vi "All Square1.vi"() -> ()   [LabVIEW 2023]
panel:
  in  "Stop 7":bool
  in  "Stop 6":bool
  in  "Stop 5":bool
  in  "Stop 4":bool
  in  "Stop 3":bool
  in  "Stop 2":bool
  in  "Start 2":bool
  in  "Start":bool
  in  "Remove 4":bool
  in  "Remove 3":bool
  in  "Remove 2":bool
  in  "Remove":bool
  in  "OK 5":bool
  in  "OK 4":bool
  in  "OK 3":bool
  in  "OK 2":bool
  in  "OK":bool
  in  "Hibernet":bool
  in  "Halt":bool
  in  "Finish 4":bool
  in  "Finish 3":bool
  in  "Finish 2":bool
  in  "Finish":bool
  in  "Exit 5":bool
  in  "Exit 4":bool
  in  "Exit 3":bool
  in  "Exit 2":bool
  in  "Exit":bool
  in  "EXE":bool
  in  "Delete 2":bool
  in  "Delete":bool
  in  "Close 4":bool
  in  "Close 3":bool
  in  "Close 2":bool
  in  "Close":bool
  in  "Clear":bool
  in  "Cancel 4":bool
  in  "Cancel 3":bool
  in  "Cancel 2":bool
  in  "Cancel":bool
  in  "Apply 7":bool
  in  "Apply 6":bool
  in  "Apply 5":bool
  in  "Apply 4":bool
  in  "Apply 3":bool
  in  "Apply 2":bool
  in  "Apply":bool
  in  "Add 6":bool
  in  "Add 5":bool
  in  "Add 4":bool
  in  "Add 3":bool
  in  "Add 2":bool
  in  "Add":bool
  in  "Stop":bool
  in  "DB_Remove":bool
  in  "DB_Comit":bool
  in  "DB_Add":bool
  in  "URL":bool
  in  "UP 7":bool
  in  "UP 6":bool
  in  "UP 5":bool
  in  "UP 4":bool
  in  "UP 3":bool
  in  "UP 2":bool
  in  "UP":bool
  in  "Undo 2":bool
  in  "Undo":bool
  in  "Top 3":bool
  in  "Top 2":bool
  in  "Top":bool
  in  "Reload 2":bool
  in  "Reload":bool
  in  "Refresh 3":bool
  in  "Refresh 2":bool
  in  "Refresh":bool
  in  "Redo 2":bool
  in  "Redo":bool
  in  "Next 8":bool
  in  "Next 7":bool
  in  "Next 6":bool
  in  "Next 5":bool
  in  "Next 4":bool
  in  "Next 3":bool
  in  "Next 2":bool
  in  "Next":bool
  in  "Exchange":bool
  in  "Down 7":bool
  in  "Down 6":bool
  in  "Down 5":bool
  in  "Down 4":bool
  in  "Down 3":bool
  in  "Down 2":bool
  in  "Down":bool
  in  "Bottom 4":bool
  in  "Bottom 3":bool
  in  "Bottom 2":bool
  in  "Bottom":bool
  in  "Back 9":bool
  in  "Back 8":bool
  in  "Back 7":bool
  in  "Back 6":bool
  in  "Back 5":bool
  in  "Back 4":bool
  in  "Back 3":bool
  in  "Back 2":bool
  in  "Back":bool
  in  "XML":bool
  in  "Word":bool
  in  "Text":bool
  in  "Sync":bool
  in  "SQL":bool
  in  "PPT":bool
  in  "PNG 2":bool
  in  "PNG":bool
  in  "Play 4":bool
  in  "PDF 4":bool
  in  "PDF 3":bool
  in  "PDF 2":bool
  in  "PDF":bool
  in  "Paint":bool
  in  "Notepad":bool
  in  "JPG":bool
  in  "JPEG 2":bool
  in  "JPEG":bool
  in  "Java":bool
  in  "Jar":bool
  in  "GIF":bool
  in  "Excel":bool
  in  "Docs":bool
  in  "CHM":bool
  in  "C++":bool
  in  "C":bool
  in  "BMP":bool
  in  "ZIP":bool
  in  "Wifi 4":bool
  in  "Wifi 3":bool
  in  "Wifi 2":bool
  in  "USB":bool
  in  "Trafic":bool
  in  "Mouse":bool
  in  "Memory":bool
  in  "Hardware":bool
  in  "Connect 2":bool
  in  "Connect":bool
  in  "Com Port":bool
  in  "Bluetooth":bool
  in  "Wifi":bool
  in  "Rewind 2":bool
  in  "Rewind":bool
  in  "Real":bool
  in  "Play 3":bool
  in  "Play 2":bool
  in  "Play":bool
  in  "Pause 4":bool
  in  "Pause 3":bool
  in  "Pause 2":bool
  in  "Pause":bool
  in  "Multimedia":bool
  in  "Game":bool
  in  "Forword 3":bool
  in  "Forword 2":bool
  in  "Forword":bool
  in  "Eject 3":bool
  in  "Eject 2":bool
  in  "Eject":bool
  in  "VLC":bool
  in  "Theme 2":bool
  in  "Theme":bool
  in  "Restore":bool
  in  "Restart":bool
  in  "Reset":bool
  in  "Info 2":bool
  in  "Info":bool
  in  "Import":bool
  in  "Help 3":bool
  in  "Help 2":bool
  in  "Help":bool
  in  "Graph 2":bool
  in  "Graph":bool
  in  "Fulscreen 2":bool
  in  "Fulscreen":bool
  in  "Folder_User":bool
  in  "Folder_System":bool
  in  "Folder_Lock":bool
  in  "Folder_Home":bool
  in  "Folder_Add":bool
  in  "Folder":bool
  in  "Filter":bool
  in  "Export":bool
  in  "Chart":bool
  in  "Burn 2":bool
  in  "Burn":bool
  in  "Warning":bool
  in  "Spellcheck 3":bool
  in  "Spellcheck 2":bool
  in  "Spellcheck":bool
  in  "Save_As 4":bool
  in  "Save_As 3":bool
  in  "Save_As 2":bool
  in  "Save_As":bool
  in  "Save_All 4":bool
  in  "Save_All 3":bool
  in  "Save_All 2":bool
  in  "Save_All":bool
  in  "Save 5":bool
  in  "Save 4":bool
  in  "Save 3":bool
  in  "Save 2":bool
  in  "Save":bool
  in  "RTF":bool
  in  "Revert 3":bool
  in  "Revert 2":bool
  in  "Revert":bool
  in  "Report 2":bool
  in  "Report":bool
  in  "Formula":bool
  in  "Font":bool
  in  "Calendar 2":bool
  in  "Calendar":bool
  in  "Calc 3":bool
  in  "Calc 2":bool
  in  "Calc":bool
  in  "Address":bool
  in  "Spreadsheet":bool
  in  "Schedule 2":bool
  in  "Clock 4":bool
  in  "Clock 3":bool
  in  "Clock 2":bool
  in  "Clock":bool
  in  "Schedule":bool
  in  "Zoomout 2":bool
  in  "ZoomIn 3":bool
  in  "ZoomIn 2":bool
  in  "ZoomIn":bool
  in  "To DO":bool
  in  "Sort":bool
  in  "Setting 3":bool
  in  "Setting 2":bool
  in  "Setting":bool
  in  "Search 2":bool
  in  "Search":bool
  in  "Repair":bool
  in  "Protect":bool
  in  "Printer_Delet":bool
  in  "Printer_Add":bool
  in  "Printer":bool
  in  "Paste 2":bool
  in  "Paste":bool
  in  "Organize":bool
  in  "Error 2":bool
  in  "Error":bool
  in  "Edit":bool
  in  "Cut 4":bool
  in  "Cut 3":bool
  in  "Cut 2":bool
  in  "Cut":bool
  in  "Copy":bool
  in  "Config 3":bool
  in  "Config 2":bool
  in  "Config":bool
  in  "Clipboard":bool
  in  "Zoomout":bool
  in  "User_Info 2":bool
  in  "User_Delete":bool
  in  "User_Add":bool
  in  "User":bool
  in  "Logout 4":bool
  in  "Logout 3":bool
  in  "Logout 2":bool
  in  "Logout":bool
  in  "Logoff":bool
  in  "LogIN 2":bool
  in  "LogIN":bool
  in  "Lock":bool
  in  "User_Info":bool
  in  "Attach":bool
  in  "Download 2":bool
  in  "Web 2":bool
  in  "Network":bool
  in  "Mail_Send":bool
  in  "Mail_Reply 2":bool
  in  "Mail_Reply":bool
  in  "Mail_Pref":bool
  in  "Mail_Imp":bool
  in  "Mail_Fwd":bool
  in  "Mail_Delete":bool
  in  "Mail":bool
  in  "Home 2":bool
  in  "History_Delete":bool
  in  "History":bool
  in  "FTP 2":bool
  in  "FTP":bool
  in  "Firefox 2":bool
  in  "Firefox":bool
  in  "Fav":bool
  in  "Download":bool
  in  "Web":bool
  in  "Home":bool
  in  "Bug":bool
  # "Action"
  # "Database"
  # "Direction"
  # "File_Format"
  # "Hardware"
  # "Media"
  # "Misc"
  # "Office"
  # "Time"
  # "Tool"
  # "User"
  # "Web"
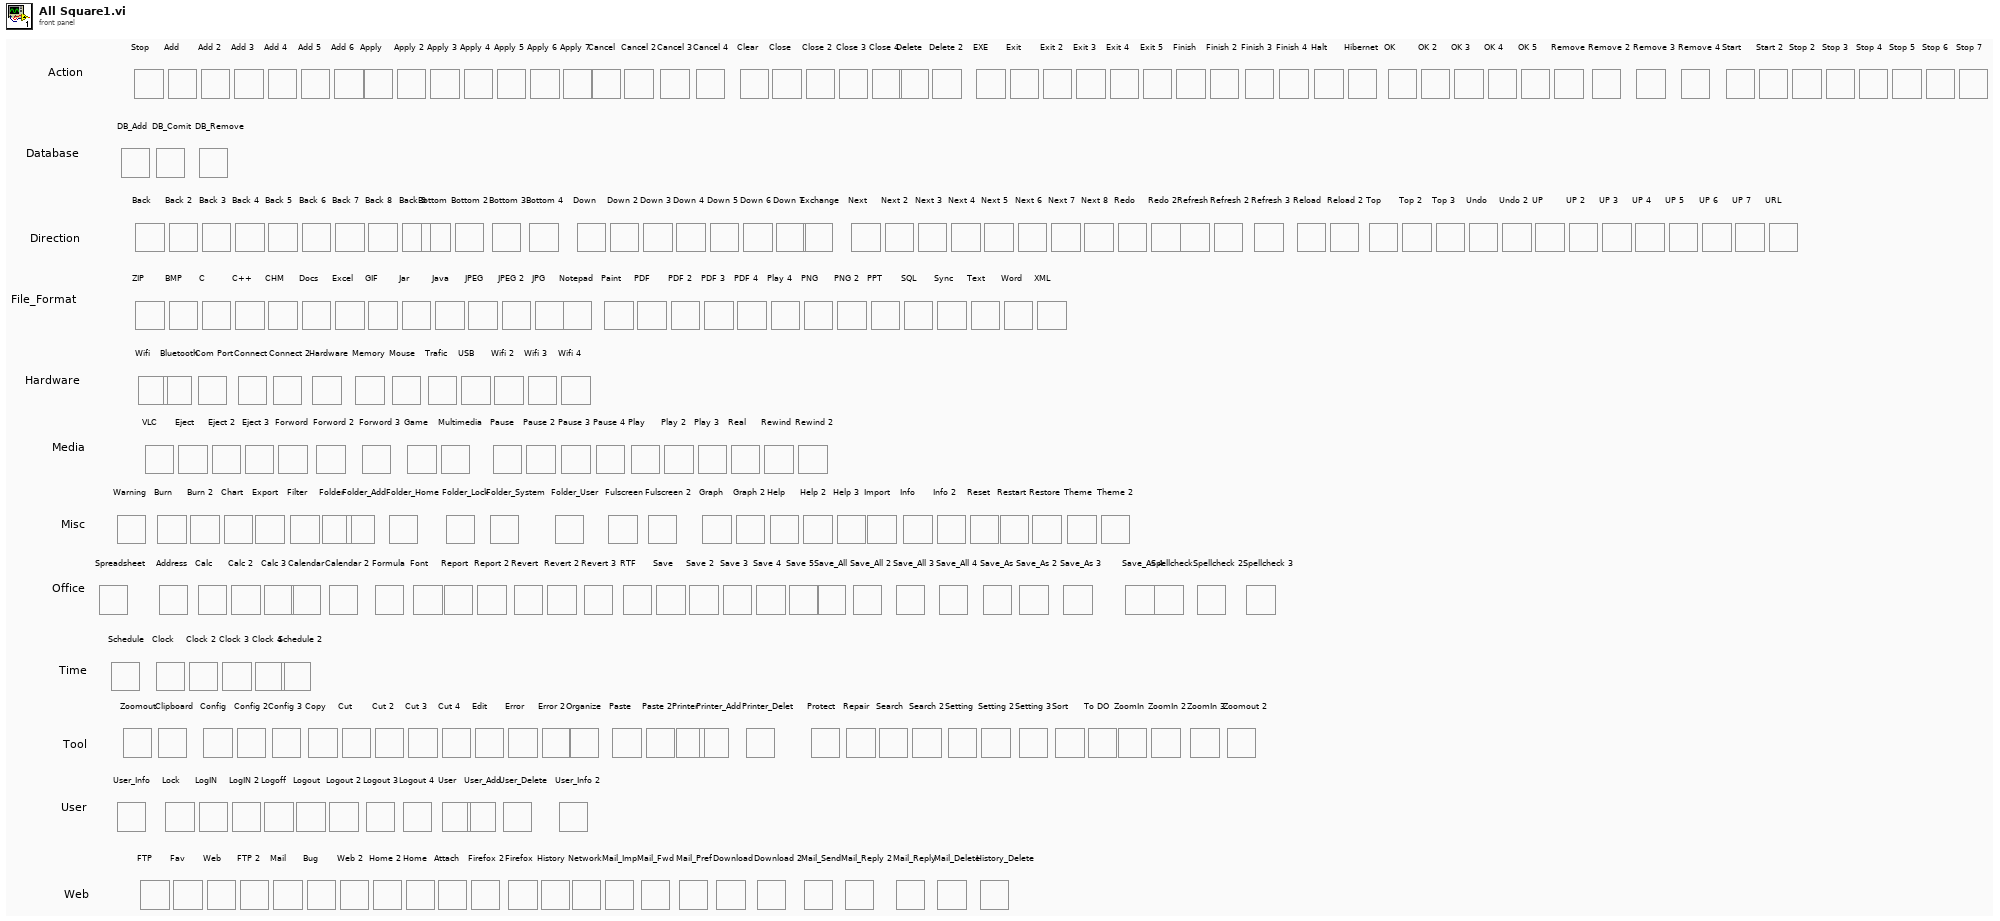
[diagram p1: front panel]
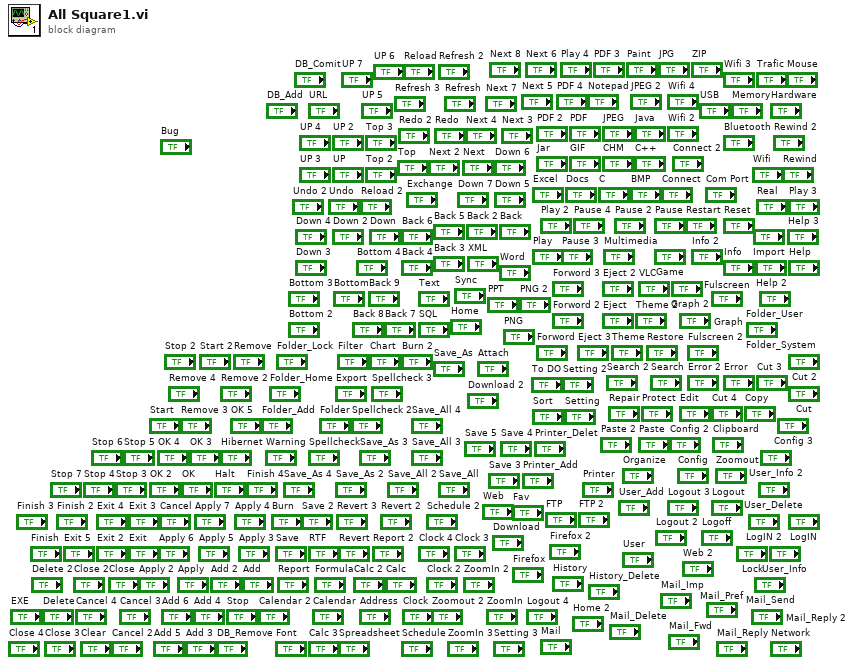
[diagram p0: block diagram]
diagram:
